vi "LatchBoolean.vi"(11 "Input":bool) -> (3 "Output":bool)   [LabVIEW 2016]
panel:
  out "Latch thing":bool
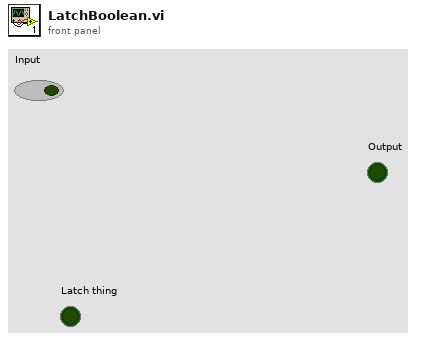
[diagram p1: front panel]
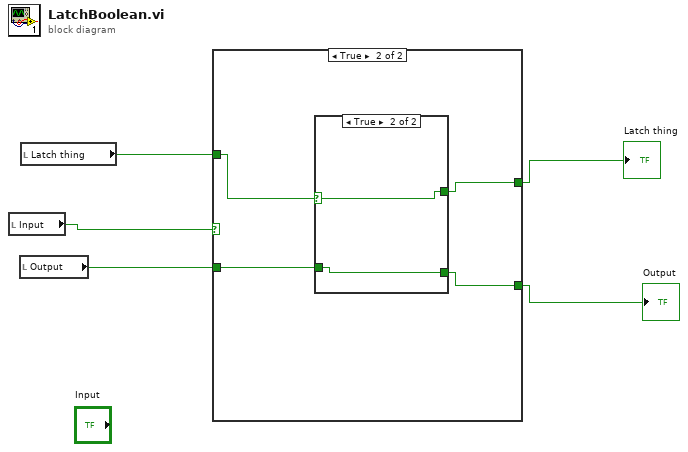
[diagram p0: block diagram]
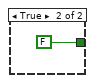
[diagram p3: hidden frame]
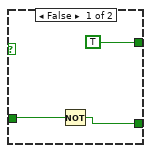
[diagram p4: hidden frame]
diagram:
  n1 = local read "Input"() -> (w5:bool)
  n2 = local read "Output"() -> (w2:bool)
  n3 = local read "Latch thing"() -> (w4:bool)
  n4 = case shown="True" w5 {
    tunnel: w4 -> [w8 w14]
    tunnel: [w7 w11] -> w3
    tunnel: w2 -> [w6 w13]
    tunnel: [w6 w12] -> w1
    frame False {
      n5 = case shown="False" w8 {
        selector: w8 -> [w9 _]
        tunnel: [w9 FALSE] -> w7
        frame False {
        }
        frame True {
        }
      }
    }
    frame True {
      n6 = case shown="True" w14 {
        selector: w14 -> [_ w18]
        tunnel: w13 -> [w17 w19]
        tunnel: [w16 w19] -> w12
        tunnel: [TRUE w18] -> w11
        frame False {
          n7 = Not(x=w17) -> (.not. x?=w16:bool)
        }
        frame True {
        }
      }
    }
  }
  "Output" <- w1
  "Latch thing" <- w3
